vi "Signal.vi"(3 "error in (no error)":errorcluster caption="错误输入（无错误）", 4 "dt":dbl, 5 "数据":fxp<+/-,24,5>[](array[numeric])) -> (0 "error out":errorcluster caption="错误输出", 1 "原始信号频谱":waveform(dbl)(graph), 2 "原始信号":waveform(dbl)(graph))   [LabVIEW 2019]
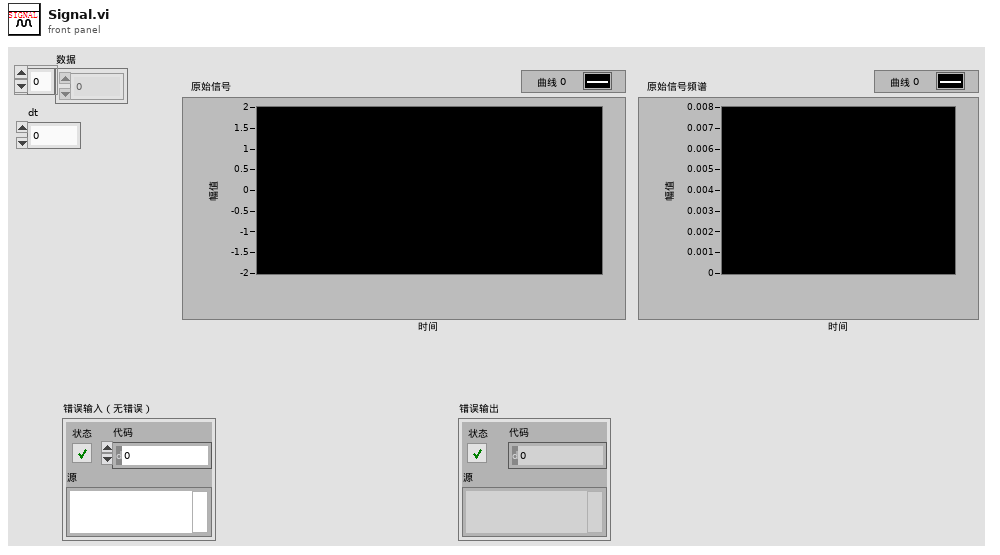
[diagram p1: front panel]
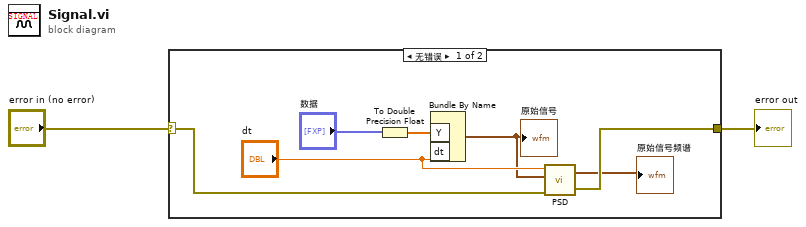
[diagram p0: block diagram]
diagram:
  n1 = case shown="无错误" "error in (no error)" {
    selector: "error in (no error)" -> [w5 w10]
    tunnel: [w4 w10] -> w1
    frame No Error {
      n2 = To Double Precision Float(number="数据") -> (double precision float=w9:dbl[])
      n3 = Bundle By Name("Y"=w9, "dt"="dt") -> (w6:waveform(dbl))  [unwired: 1 in]
      "原始信号" <- w6
      n4 = call "PSD.vi"("error in (no error)"=w5, "输入波形"=w6, "dt"="dt") -> ("error out"=w4:errorcluster, "波形图"=→"原始信号频谱":waveform(dbl))  [unwired: 3 in]
    }
    frame Error {
    }
  }
  "error out" <- w1
